vi "LVObject to JSON - 200 Elements No Pretty Print - Produces Regular Output.vi"() -> ()   [LabVIEW 2017, in "Tests.lvlib" / "Pretty Print.lvlib"]
uses:
  Pretty Print.lvlib
  Flatten To JSON Object/Flatten To JSON Object.lvclass
  Strings/Strings.lvclass
  <vilib>/addons/_JKI Toolkits/Caraya/classes/Assert/Assert Equal Value_Variant.vi
  <vilib>/addons/_JKI Toolkits/Caraya/classes/Test/Test.lvclass
  <vilib>/addons/_JKI Toolkits/Caraya/classes/Assert/Assert.lvclass
panel:
  out "error out":errorcluster
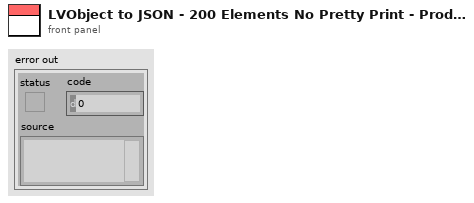
[diagram p1: front panel]
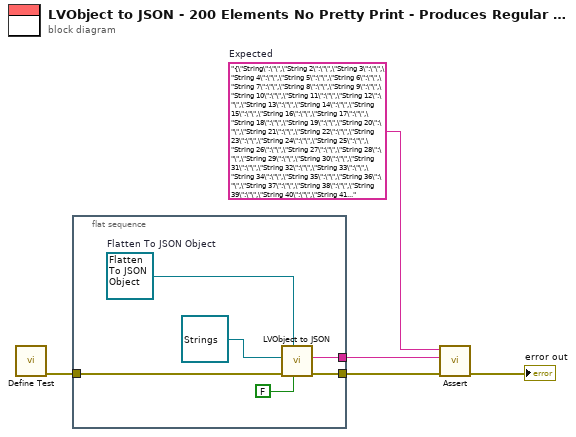
[diagram p0: block diagram]
diagram:
  w1 = "{\"String\":\"\",\"String 2\":\"\",\"String 3\":\"\",\"String 4\":\"\",\"String 5\":\"\",\"String 6\":\"\",\"String 7\":\"\",\"String 8\":\"\",\"String 9\":\"\",\"String 10\":\"\",\"String 11\":\"\",\"String 12\":\"\",\"String 13\":\"\",\"String 14\":\"\",\"String 15\":\"\",\"String 16\":\"\",\"String 17\":\"\",\"String 18\":\"\",\"String 19\":\"\",\"String 20\":\"\",\"String 21\":\"\",\"String 22\":\"\",\"String 23\":\"\",\"String 24\":\"\",\"String 25\":\"\",\"String 26\":\"\",\"String 27\":\"\",\"String 28\":\"\",\"String 29\":\"\",\"String 30\":\"\",\"String 31\":\"\",\"String 32\":\"\",\"String 33\":\"\",\"String 34\":\"\",\"String 35\":\"\",\"String 36\":\"\",\"String 37\":\"\",\"String 38\":\"\",\"String 39\":\"\",\"String 40\":\"\",\"String 41\":\"\",\"String 42\":\"\",\"String 43\":\"\",\"String 44\":\"\",\"String 45\":\"\",\"String 46\":\"\",\"String 47\":\"\",\"String 48\":\"\",\"String 49\":\"\",\"String 50\":\"\",\"String 51\":\"\",\"String 52\":\"\",\"String 53\":\"\",\"String 54\":\"\",\"String 55\":\"\",\"String 56\":\"\",\"String 57\":\"\",\"String 58\":\"\",\"String 59\":\"\",\"String 60\":\"\",\"String 61\":\"\",\"String 62\":\"\",\"String 63\":\"\",\"String 64\":\"\",\"String 65\":\"\",\"String 66\":\"\",\"String 67\":\"\",\"String 68\":\"\",\"String 69\":\"\",\"String 70\":\"\",\"String 71\":\"\",\"String 72\":\"\",\"String 73\":\"\",\"String 74\":\"\",\"String 75\":\"\",\"String 76\":\"\",\"String 77\":\"\",\"String 78\":\"\",\"String 79\":\"\",\"String 80\":\"\",\"String 81\":\"\",\"String 82\":\"\",\"String 83\":\"\",\"String 84\":\"\",\"String 85\":\"\",\"String 86\":\"\",\"String 87\":\"\",\"String 88\":\"\",\"String 89\":\"\",\"String 90\":\"\",\"String 91\":\"\",\"String 92\":\"\",\"String 93\":\"\",\"String 94\":\"\",\"String 95\":\"\",\"String 96\":\"\",\"String 97\":\"\",\"String 98\":\"\",\"String 99\":\"\",\"String 100\":\"\",\"String 101\":\"\",\"String 102\":\"\",\"String 103\":\"\",\"String 104\":\"\",\"String 105\":\"\",\"String 106\":\"\",\"String 107\":\"\",\"String 108\":\"\",\"String 109\":\"\",\"String 110\":\"\",\"String 111\":\"\",\"String 112\":\"\",\"String 113\":\"\",\"String 114\":\"\",\"String 115\":\"\",\"String 116\":\"\",\"String 117\":\"\",\"String 118\":\"\",\"String 119\":\"\",\"String 120\":\"\",\"String 121\":\"\",\"String 122\":\"\",\"String 123\":\"\",\"String 124\":\"\",\"String 125\":\"\",\"String 126\":\"\",\"String 127\":\"\",\"String 128\":\"\",\"String 129\":\"\",\"String 130\":\"\",\"String 131\":\"\",\"String 132\":\"\",\"String 133\":\"\",\"String 134\":\"\",\"String 135\":\"\",\"String 136\":\"\",\"String 137\":\"\",\"String 138\":\"\",\"String 139\":\"\",\"String 140\":\"\",\"String 141\":\"\",\"String 142\":\"\",\"String 143\":\"\",\"String 144\":\"\",\"String 145\":\"\",\"String 146\":\"\",\"String 147\":\"\",\"String 148\":\"\",\"String 149\":\"\",\"String 150\":\"\",\"String 151\":\"\",\"String 152\":\"\",\"String 153\":\"\",\"String 154\":\"\",\"String 155\":\"\",\"String 156\":\"\",\"String 157\":\"\",\"String 158\":\"\",\"String 159\":\"\",\"String 160\":\"\",\"String 161\":\"\",\"String 162\":\"\",\"String 163\":\"\",\"String 164\":\"\",\"String 165\":\"\",\"String 166\":\"\",\"String 167\":\"\",\"String 168\":\"\",\"String 169\":\"\",\"String 170\":\"\",\"String 171\":\"\",\"String 172\":\"\",\"String 173\":\"\",\"String 174\":\"\",\"String 175\":\"\",\"String 176\":\"\",\"String 177\":\"\",\"String 178\":\"\",\"String 179\":\"\",\"String 180\":\"\",\"String 181\":\"\",\"String 182\":\"\",\"String 183\":\"\",\"String 184\":\"\",\"String 185\":\"\",\"String 186\":\"\",\"String 187\":\"\",\"String 188\":\"\",\"String 189\":\"\",\"String 190\":\"\",\"String 191\":\"\",\"String 192\":\"\",\"String 193\":\"\",\"String 194\":\"\",\"String 195\":\"\",\"String 196\":\"\",\"String 197\":\"\",\"String 198\":\"\",\"String 199\":\"\",\"String 200\":\"\"}"  # Expected
  n1 = call <vilib>:"Define Test.vi"() -> ("error out"=w4:errorcluster)  [unwired: 11 in]
  n2 = flat-sequence {
    tunnel: w4 -> [w8]
    tunnel: [w10] -> w3
    tunnel: [w9] -> w2
    frame #0 {
      w11 = refnum<class "Flatten To JSON Object.lvclass"> refnum  # Flatten To JSON Object
      n3 = call-dynamic "LVObject to JSON.vi"("Pretty Print?"=FALSE, "LVClass Serializer"=w11, "error in (no error)"=w8, "Object"=refnum<class "Strings.lvclass"> refnum ("Tests.lvlib:Strings.lvclass")) -> ("error out"=w10:errorcluster, "<JSON>Object"=w9:string)  [unwired: 6 in]
    }
  }
  n4 = call-poly <vilib>:"Assert.vi"("error in (no error)"=w3, "Y"=w2, "X"=w1) -> ("error out"=→"error out":errorcluster)  [unwired: 8 in]
